vi "SMO.Example.SetData.vi"(8 "error in (no error)":errorcluster, 9 "Flow 2":dbl, 10 "Flow 1":dbl, 11 "SMO.Example":refnum<class "SMO.Example.lvclass">) -> (0 "error out":errorcluster, 3 "SMO.Example out":refnum<class "SMO.Example.lvclass">)   [LabVIEW 2013, in "SMO.Example.lvclass"]
doc: "---------------------------------------------------------------\nJKI State Machine Objects™\nhttp://jki.net/state-machine-objects/\nCopyright (C) 2005-2015, JKI <info@jki.net>\nALL RIGHTS RESERVED"
uses:
  SMO.Example.lvclass
  Typedefs/DataChanged--EventData--Cluster.ctl
  SMO.Example.lvclass/SMO.Example.ctl
panel:
  # "For instructions on how to use the JKI State Machine Objects, examples and video tutorials, visit:\nhttp://jki.net/state-machine-objects/\n\nJKI State Machine Objects™\nhttp://jki.net/state-machine-objects/\nCopyright (C) 2005-2015, JKI <info@jki.net>\nALL RIGHTS RESERVED"
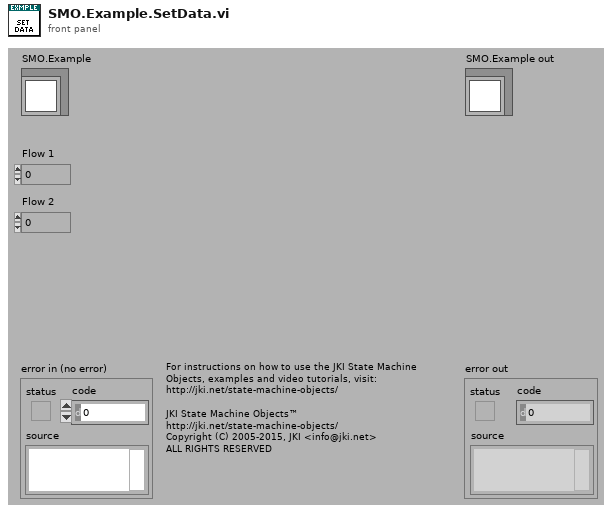
[diagram p1: front panel]
types:
  T1 = typedef "SMO.Example.lvclass/DataChanged--EventData--Cluster.ctl" = cluster{"Timestamp":timestamp, "Flow 1":dbl, "Flow 2":dbl}
  T2 = typedef "SMO.Example.lvclass/PrivateData--Ref.ctl" = refnum<data-value>
  T3 = typedef "SMO.Example.lvclass/PrivateData--Cluster.ctl" = cluster{"Configuration":T4, "Public Events":T5, "Protected Events":T6, "Flow 1":dbl, "Flow 2":dbl}
  T4 = typedef "SMO.Example.lvclass/Configuration--Cluster.ctl" = cluster{"Suffix":string}
  T5 = typedef "SMO.Example.lvclass/PublicEvents--Cluster.ctl" = cluster{"Data Changed":refnum<user-event>}
  T6 = typedef "SMO.Example.lvclass/ProtectedEvents--Cluster.ctl" = cluster{"API_Template":refnum<user-event>, "PumpState":refnum<user-event>, "Valve State":refnum<user-event>}
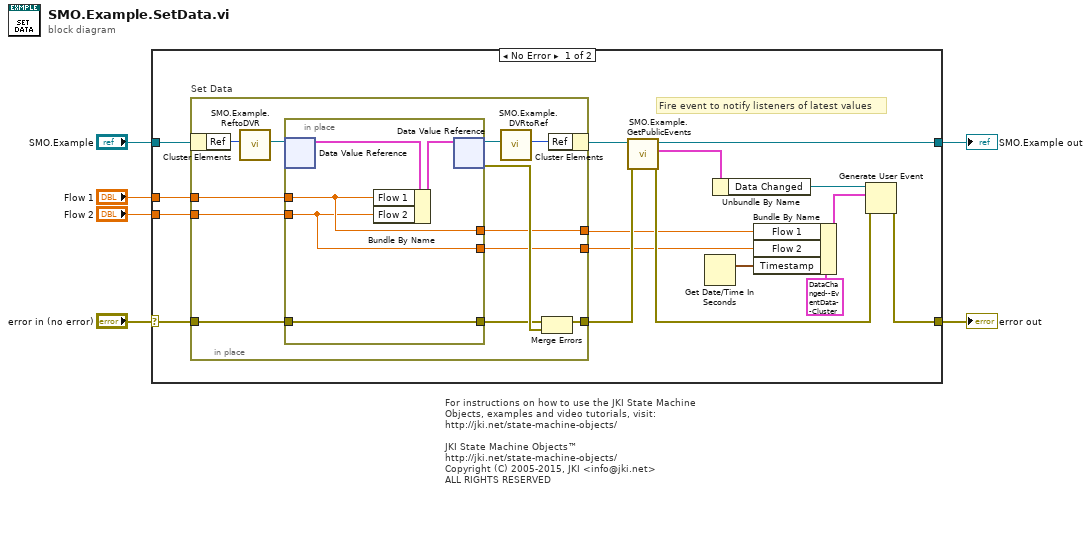
[diagram p0: block diagram]
diagram:
  # "For instructions on how to use the JKI State Machine Objects, examples and video tutorials, visit:\nhttp://jki.net/state-machine-objects/\n\nJKI State Machine Objects™\nhttp://jki.net/state-machine-objects/\nCopyright (C) 2005-2015, JKI <info@jki.net>\nALL RIGHTS RESERVED"
  n1 = case shown="No Error" "error in (no error)" {
    selector: "error in (no error)" -> [w20 w40]
    tunnel: "SMO.Example" -> [w21 w41]
    tunnel: [w10 w40] -> w5
    tunnel: [w18 w41] -> w4
    tunnel: "Flow 1" -> [w22 _]
    tunnel: "Flow 2" -> [w9 _]
    frame No Error {
      # "Fire event to notify listeners of latest values"
      n2 = in-place "Set Data" {
        in-place-border: w20 -> [w34]
        in-place-border: [w31] -> w17
        in-place-border: w22 -> [w30]
        in-place-border: [w29] -> w8
        in-place-border: w9 -> [w28]
        in-place-border: [w27] -> w7
        n3 = in-place-cluster #1(w21) -> ("Ref"=w26:u32)
        n4 = call "SMO.Example.ReftoDVR.vi"("Ref"=w26) -> ("Ref"=w25:T2)  [unwired: 10 in]
        n5 = in-place {
          in-place-border: w34 -> [w39]
          in-place-border: [w39] -> w32
          in-place-border: w30 -> [w37]
          in-place-border: [w37] -> w29
          in-place-border: w28 -> [w35]
          in-place-border: [w35] -> w27
          n6 = in-place-dvr #2(w25) -> (w36:T3)  [unwired: 1 out]
          n7 = Bundle By Name(cluster=w36, "Flow 1"=w37, "Flow 2"=w35) -> (w38:T3)
          n8 = in-place-dvr #2(w38) -> (w24:T2, w33:errorcluster)
        }
        n9 = call "SMO.Example.DVRtoRef.vi"("Ref"=w24) -> ("Ref"=w23:u32)  [unwired: 10 in]
        n10 = Merge Errors(w32, w33) -> (w31:errorcluster)
        n11 = in-place-cluster #1("Ref"=w23) -> (w19:refnum<class "SMO.Example.lvclass">)
      }
      n12 = call "SMO.Example.GetPublicEvents.vi"("error in (no error)"=w17, "SMO.Example"=w19) -> ("error out"=w11:errorcluster, "Public Events"=w16:T5, "SMO.Example out"=w18:refnum<class "SMO.Example.lvclass">)  [unwired: 7 in]
      n13 = Get Date/Time In Seconds() -> (seconds since 1Jan1904=w12:timestamp)
      n14 = Unbundle By Name(w16) -> ("Data Changed"=w15:refnum<user-event>)
      n15 = Bundle By Name(cluster=T1 {"Timestamp"=timestamp(0 s since 1904-01-01), "Flow 1"=0.0, "Flow 2"=0.0} ("event data"), "Flow 1"=w8, "Flow 2"=w7, "Timestamp"=w12) -> (w13:T1)
      n16 = Generate User Event(user event=w15, event data cluster=w13, error in=w11) -> (error out=w10:errorcluster)  [unwired: 1 in, 1 out]
    }
    frame Error {
    }
  }
  "error out" <- w5
  "SMO.Example out" <- w4
